vi "DHE_DRV_read_memory.vi"(0 "fd":i32, 5 "type":string, 7 "address":i32, 11 "error in (no error)":errorcluster) -> (4 "fd":i32, 8 "return value":i32, 15 "error out":errorcluster)   [LabVIEW 2016]
doc: "This VI closes the I/O interface with the instrument."
uses:
  c/lib/libarcDHE.so
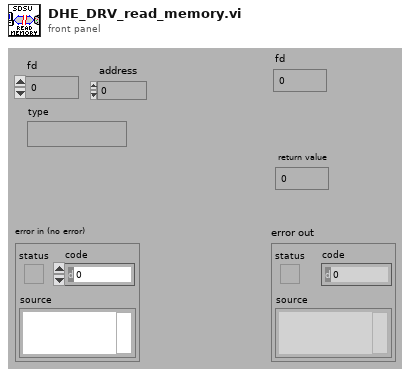
[diagram p1: front panel]
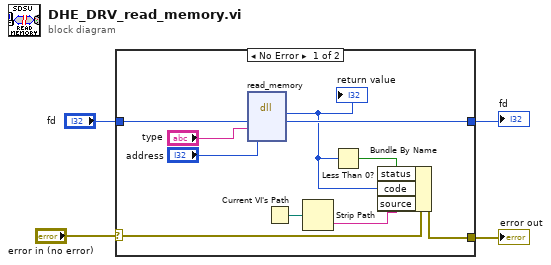
[diagram p0: block diagram]
diagram:
  n1 = case shown="No Error" "error in (no error)" {
    selector: "error in (no error)" -> [w5 w15]
    tunnel: "fd" -> [w14 w16]
    tunnel: [w8 w16] -> w3
    tunnel: [w7 w15] -> w2
    frame No Error {
      n2 = dll-call lib="home/simager/panview/PAN/Modules/SDSU/private/c/lib/libarcDHE.so" fn="read_memory"("fd"=w14, "type"="type", "address"="address") -> (w6:i32, "fd"=w8:i32)  [unwired: 5 in, 2 out]
      "return value" <- w6
      n3 = Current VI's Path() -> (path=w12:path)
      n4 = Strip Path(path=w12) -> (name=w11:string)  [unwired: 1 out]
      n5 = Less Than 0?(x=w6) -> (x < 0?=w13:bool)
      n6 = Bundle By Name(cluster=w5, "status"=w13, "code"=w6, "source"=w11) -> (w7:errorcluster)
    }
    frame Error {
    }
  }
  "error out" <- w2
  "fd" <- w3
